vi "Convert activity to string.vi"(4 "Activity log In":T1 {"Epoch sec" format="%.2e"}) -> (1 "Activity log string":string)   [LabVIEW 2013]
doc: "Converts Activity Log from array of cluster into a string. String has a carriage return - line feed for each activity in array."
uses:
  User Access Type defs/Acitivity cluster array.ctl
  User Access Type defs/Acitivity cluster.ctl
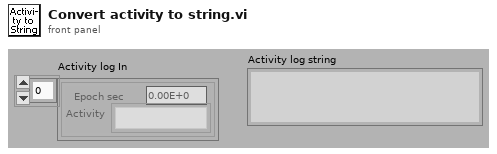
[diagram p1: front panel]
types:
  T1 = typedef "Acitivity cluster array.ctl" = T2[]
  T2 = typedef "Acitivity cluster.ctl" = cluster{"Epoch sec":dbl, "Activity":string}
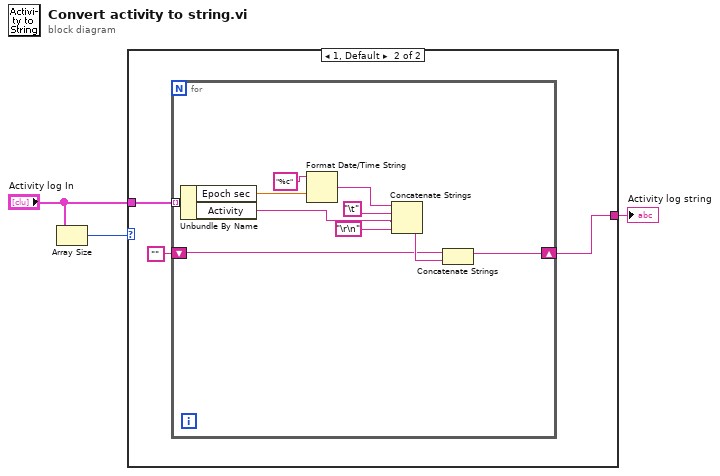
[diagram p0: block diagram]
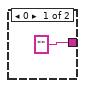
[diagram p2: hidden frame]
diagram:
  n1 = Array Size(array="Activity log In") -> (size(s)=w2:i32)
  n2 = case shown="1, Default" w2 {
    tunnel: "Activity log In" -> [_ w7]
    tunnel: ["" ("date/time string") w6] -> w1
    frame 0 {
    }
    frame 1, Default {
      n3 = for {
        tunnel: w7 -> [w17] mode=indexing
        shift-right: [w13] -> w6
        shift-left: "" ("date/time string") -> [w11]
        n4 = Unbundle By Name(w17) -> ("Epoch sec"=w10:dbl, "Activity"=w8:string)
        n5 = Format Date/Time String(time format string (%c)="%c", seconds (now)=w10) -> (date/time string=w9:string)  [unwired: 1 out]
        n6 = Concatenate Strings(w9, "\t", w8, "\r\n") -> (w12:string)
        n7 = Concatenate Strings(w11, w12) -> (w13:string)
      }
    }
  }
  "Activity log string" <- w1
